vi "from string 1.0.vi"(8 "error in (no error)":errorcluster, 10 "data":string, 11 "UI Reference configuration in":refnum<class "UI Reference configuration.lvclass">) -> (0 "error out":errorcluster, 3 "UI Reference configuration out":refnum<class "UI Reference configuration.lvclass">)   [LabVIEW 2015, in "UI Reference configuration.lvclass"]
uses:
  UI Reference configuration.lvclass
  <vilib>/NI/Tag Bus Module Framework/channel/TBM channel.lvclass
  Line.ctl
  UI Reference configuration.lvclass/UI Reference configuration.ctl
  <vilib>/NI/Configuration Framework/serializable configuration/NISE_CEF_serializable configuration.lvclass
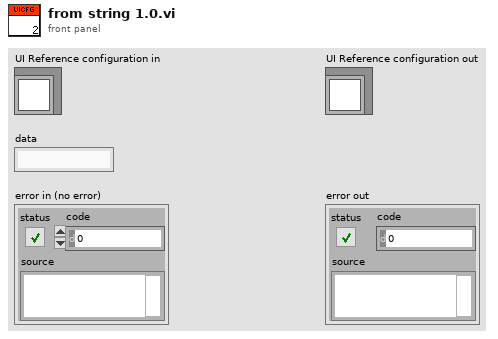
[diagram p1: front panel]
types:
  T1 = typedef "UI Reference configuration.lvclass/Line.ctl" = cluster{"channel":refnum<class "TBM channel.lvclass">}
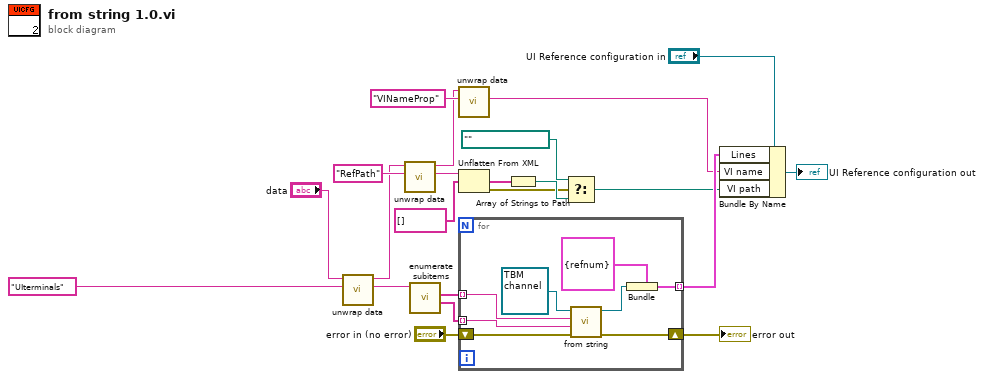
[diagram p0: block diagram]
diagram:
  n1 = call <vilib>:"unwrap data.vi"("identifier"="UIterminals", "data to unwrap"="data") -> ("unwrapped data"=w20:string, "remaining string"=w1:string)  [unwired: 8 in]
  n2 = call <vilib>:"unwrap data.vi"("identifier"="RefPath" ("additional identifier"), "data to unwrap"=w1) -> ("unwrapped data"=w9:string, "remaining string"=w11:string)  [unwired: 8 in]
  n3 = call <vilib>:"enumerate subitems.vi"("data to enumerate"=w20) -> ("associated data"=w18:string[], "discovered subitems"=w17:string[])  [unwired: 8 in, 1 out]
  n4 = call <vilib>:"unwrap data.vi"("identifier"="VINameProp" ("additional identifier"), "data to unwrap"=w11) -> ("unwrapped data"=w3:string)  [unwired: 8 in, 1 out]
  n5 = Unflatten From XML(xml string=w9, type=string[] [] ("array of strings")) -> (value=w7:string[], error out=w5:errorcluster)  [unwired: 1 in]
  n6 = for {
    shift-right: [w30] -> w22
    shift-left: "error in (no error)" -> [w29]
    tunnel: w17 -> [w28] mode=indexing
    tunnel: w18 -> [w27] mode=indexing
    tunnel: [w23] -> w21 mode=indexing
    n7 = call-dynamic "from string.vi"("error in"=w29, "channel data"=w27, "identifier"=w28, "channel in"=refnum<class "TBM channel.lvclass"> refnum) -> ("error out"=w30:errorcluster, "channel out"=w24:refnum<class "TBM channel.lvclass">)  [unwired: 6 in]
    n8 = Bundle(cluster=T1 {"channel"=refnum} ("Line"), "channel"=w24) -> (w23:T1)
  }
  "error out" <- w22
  n9 = Array of Strings to Path(0:w7) -> (2:w6:path)  [unwired: 1 in]
  n10 = Select(t=path "", s=w5, f=w6) -> (s? t:f=w2:path)
  n11 = Bundle By Name(cluster="UI Reference configuration in", "Lines"=w21, "VI name"=w3, "VI path"=w2) -> (→"UI Reference configuration out":refnum<class "UI Reference configuration.lvclass">)
